vi "Look left.vi"(8 "column":i32, 9 "row":i32, 10 "Tree":T1, 11 "Array":T1[][](array[typedef])) -> (2 "output cluster":T1)   [LabVIEW 2020]
uses:
  tree--cluster.ctl
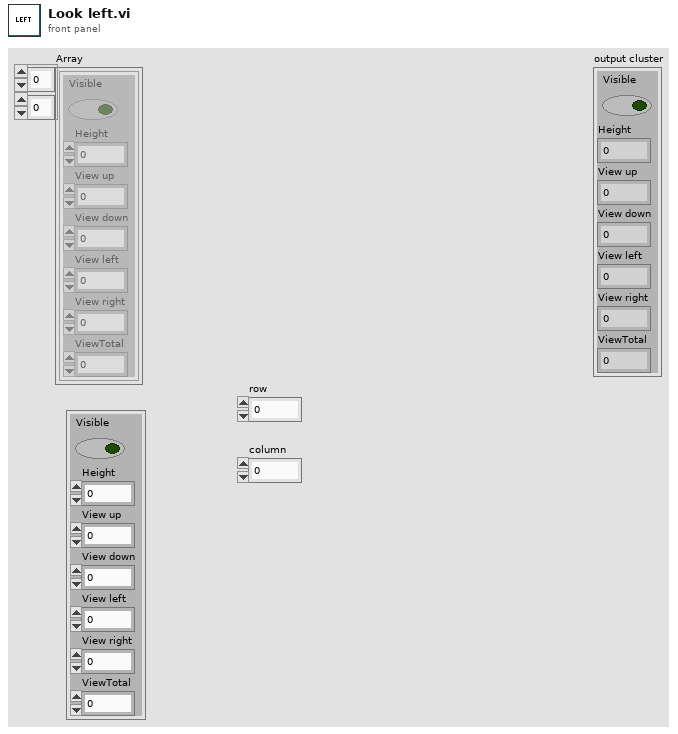
[diagram p1: front panel]
types:
  T1 = typedef "tree--cluster.ctl" = cluster{"Visible":bool, "Height":i32, "View up":i32, "View down":i32, "View left":i32, "View right":i32, "ViewTotal":i32}
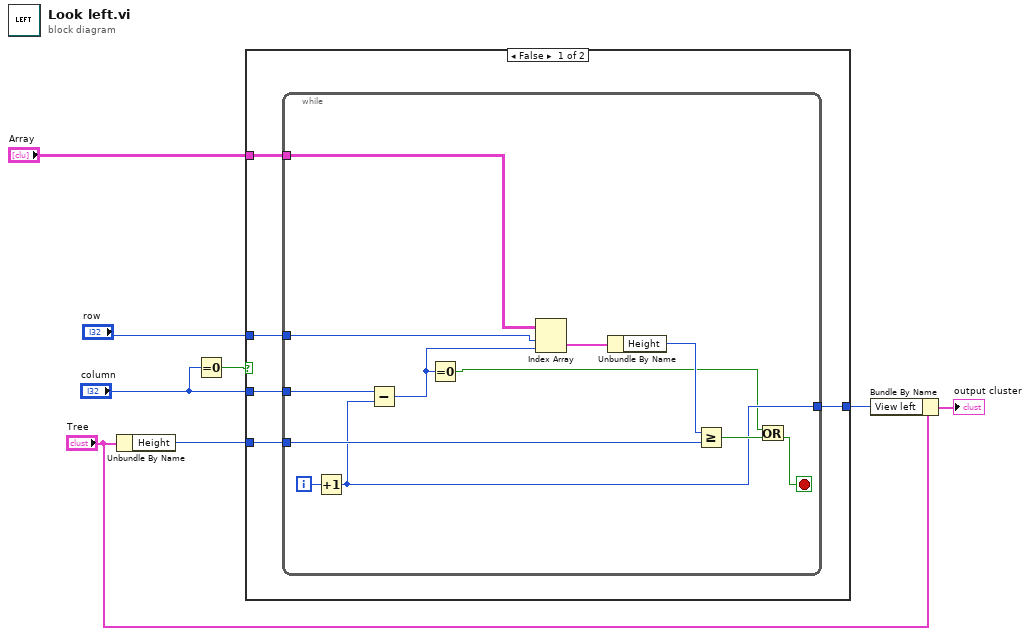
[diagram p0: block diagram]
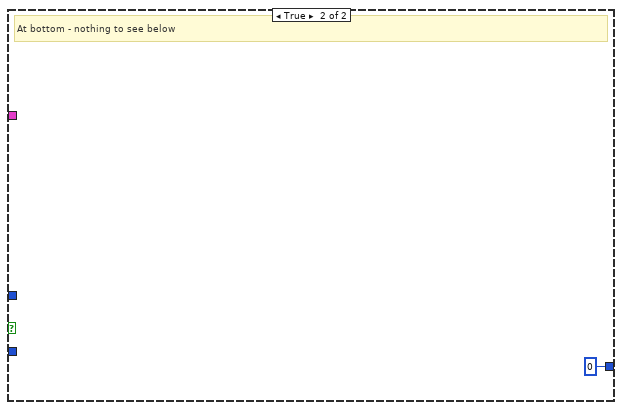
[diagram p2: hidden frame]
diagram:
  n1 = Unbundle By Name("Tree") -> ("Height"=w8:i32)
  n2 = Equal To 0?(x="column") -> (x = 0?=w2:bool)
  n3 = case shown="False" w2 {
    tunnel: w8 -> [w13 _]
    tunnel: "column" -> [w12 _]
    tunnel: "row" -> [w11 _]
    tunnel: [w10 0] -> w6
    tunnel: "Array" -> [w9 _]
    frame False {
      n4 = while {
        tunnel: w13 -> [w21]
        tunnel: w9 -> [w25]
        tunnel: w12 -> [w16]
        tunnel: w11 -> [w14]
        tunnel: [w19] -> w10
        i -> [w24]
        stop <- w18 stop-if-true
        n5 = Increment(x=w24) -> (x+1=w19:i32)
        n6 = Subtract(x=w16, y=w19) -> (x-y=w15:i32)
        n7 = Equal To 0?(x=w15) -> (x = 0?=w17:bool)
        n8 = Index Array(array=w25, index (row)=w14, index (col)=w15) -> (element=w23:T1)
        n9 = Unbundle By Name(w23) -> ("Height"=w22:i32)
        n10 = Greater Or Equal?(x=w22, y=w21) -> (x >= y?=w20:bool)
        n11 = Or(x=w17, y=w20) -> (x .or. y?=w18:bool)
      }
    }
    frame True {
      # "At bottom - nothing to see below"
    }
  }
  n12 = Bundle By Name(cluster="Tree", "View left"=w6) -> (→"output cluster":T1)
